vi "趋势图对话框.vi"(9 "参数":string, 10 "DigNum引用句柄":refnum<vi>, 11 "原点":T1 caption="点") -> ()   [LabVIEW 2016, in "多参数状态显示.xctl"]
uses:
  <vilib>/Utility/miscctls.llb/LVPointTypeDef.ctl
panel:
  out "波形图表":dbl(graph)
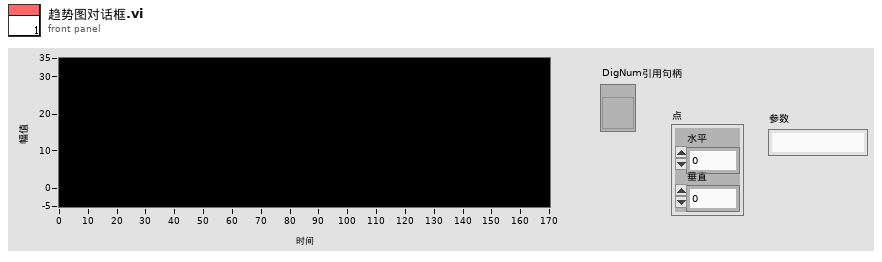
[diagram p1: front panel]
types:
  T1 = typedef "LVPointTypeDef.ctl" = cluster{"Horizontal":i16, "Vertical":i16}
  T2 = typedef "LVRectTypeDef.ctl" = cluster{"Left":i16, "Top":i16, "Right":i16, "Bottom":i16}
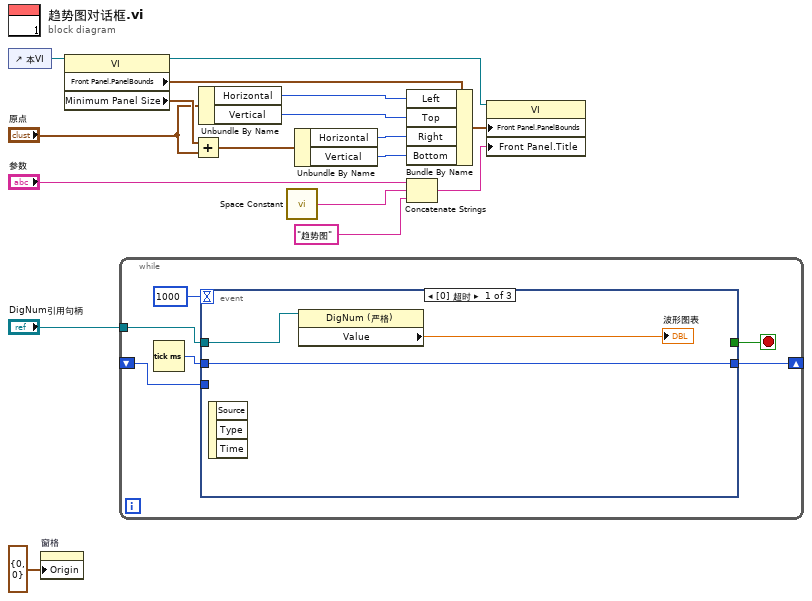
[diagram p0: block diagram]
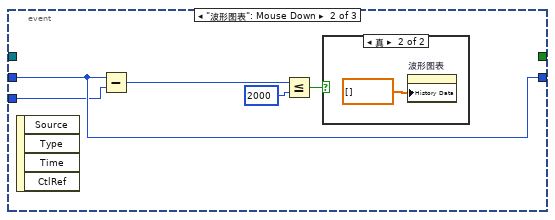
[diagram p2: hidden frame]
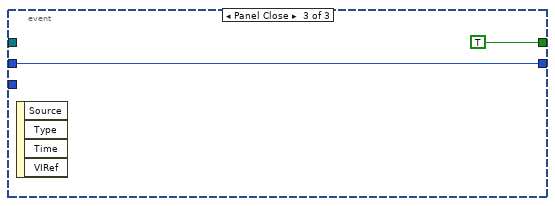
[diagram p4: hidden frame]
diagram:
  n1 = control-ref of="本VI"() -> (w16:refnum<vi>)
  n2 = property on="窗格" class="Pane"("Origin"=T1 {"Horizontal"=0, "Vertical"=0} ("原点")) -> ()  [unwired: 2 in, 2 out]
  n3 = property class="VI"(reference=w16) -> (reference out=w15:refnum<vi>, "Front Panel.PanelBounds"=w14:T2, "Minimum Panel Size"=w10:T1)  [unwired: 1 in, 1 out]
  n4 = while {
    tunnel: "DigNum引用句柄" -> [w21]
    shift-right: [w19] -> _
    shift-left: _ -> [w18]
    stop <- w23 stop-if-true
    n5 = Tick Count (ms)() -> (millisecond timer value=w20:u32)
    n6 = event shown="[0] 超时" {
      selector: _ -> [_ _ _]
      dyn-events: _ -> [_ _ _]
      timeout: 1000 -> [_ _ _]
      tunnel: [_ _ TRUE] -> w23
      tunnel: w21 -> [w26 _ _]
      tunnel: w20 -> [w25 w31 w33]
      tunnel: [w25 w31 w33] -> w19
      tunnel: w18 -> [_ w30 _]
      event Timeout {
        n7 = event-data() -> ()  [unwired: 1 in, 3 out]
        n8 = property class="DigNum (严格)"(reference=w26) -> ("Value"=→"波形图表":dbl)  [unwired: 1 in, 2 out]
      }
      event "波形图表": Mouse Down {
        n9 = event-data() -> ()  [unwired: 1 in, 4 out]
        n10 = Subtract(x=w31, y=w30) -> (x-y=w29:u32)
        n11 = Less Or Equal?(x=w29, y=u32 2000) -> (x <= y?=w27:bool)
        n12 = case shown="真" w27 {
          frame False {
          }
          frame True {
            n13 = property on="波形图表" class="WFChart (严格)"("History Data"=dbl[] [] ("历史数据")) -> ()  [unwired: 2 in, 2 out]
          }
        }
      }
      event Panel Close {
        n14 = event-data() -> ()  [unwired: 1 in, 4 out]
      }
    }
  }
  n15 = Add(x=w10, y="原点") -> (x+y=w8:T1)
  n16 = Unbundle By Name("原点") -> ("Horizontal"=w12:i16, "Vertical"=w11:i16)
  n17 = call <vilib>:"Space Constant.vi"() -> ("String"=w2:string)
  n18 = Unbundle By Name(w8) -> ("Horizontal"=w7:i16, "Vertical"=w6:i16)
  n19 = Bundle By Name(cluster=w14, "Left"=w12, "Top"=w11, "Right"=w7, "Bottom"=w6) -> (w13:T2)
  n20 = Concatenate Strings("参数", w2, "趋势图" ("字符串")) -> (w4:string)
  n21 = property class="VI"(reference=w15, "Front Panel.PanelBounds"=w13, "Front Panel.Title"=w4) -> ()  [unwired: 1 in, 2 out]
